vi "UMLEditor Main.vi"(1 "StartProject":string, 3 "StartTarget":string) -> ()   [LabVIEW 2012] (continued)
            n1875 = call <resource>:"UMLEditor getDiagramInfo.vi"("localVariables"=w4885, "error in (no error)"=w4887) -> ("saveDir"=w4893:path, "error out"=w4886:errorcluster)  [unwired: 16 out]
            n1876 = File Dialog(6:"*.txt" ("pattern"), 7:"Select script file to start executing" ("prompt"), 11:w4893) -> (1:w4890:bool, 2:w4891:bool, 3:w4888:path)  [unwired: 1 in, 4 out]
            n1877 = Compound Arithmetic op=AND(w4891, invert w4890) -> (invert w4889:bool)
          }
          frame Default {
            n1878 = Equal?(x=w4902, y=UMLEditor_statesType."ExecuteCommand" ("state")) -> (x = y?=w4901:bool)
            n1879 = call <resource>:"UMLEditor createWizardScriptFile.vi"("localVariables"=w4899, "OnlySelectedNode(False)"=w4901, "error in (no error)"=w4904) -> ("localVariables"=w4898:T7, "pathToScriptFile"=w4903:path, "Cancelled"=w4895:bool, "error out"=w4897:errorcluster)  [unwired: 13 out]
          }
        }
        n1880 = call <resource>:"CommonVIs_UmlOpenVIRef.vi"("error in"=w4879) -> ("error out"=w4873:errorcluster, "ProjectNameOut"=w4870:string)  [unwired: 3 in, 6 out]
        n1881 = call <resource>:"GDSProject_GetProjects.vi"("GetProjectRefByName"=w4870, "error in (no error)"=w4873) -> ("Projects"=w4872:string[], "Project Refnum"=w4869:refnum<vi>)  [unwired: 1 in, 15 out]
        n1882 = Search 1D Array(1D array=w4872, element=w4870) -> (index of element=w4871:i32)  [unwired: 1 out]
        n1883 = property on="Project" class="Ring (strict)"("Strings []"=w4872, "Value"=w4871) -> ()  [unwired: 2 in, 2 out]
        n1884 = property class="Project"(reference=w4869) -> (reference out=w4866:refnum<vi>, error out=w4867:errorcluster, "Path"=w4865:path)  [unwired: 1 in]
        n1885 = call <resource>:"GetRelativePathOption.vi"() -> ("UseProjectFolderAsBasePath"=w4868:bool)  [unwired: 1 in, 18 out]
        n1886 = Strip Path(path=w4865) -> (stripped path=w4862:path)  [unwired: 1 out]
        n1887 = Close Reference(reference=w4866, error in (no error)=w4867) -> (error out=w4861:errorcluster)
        n1888 = call <resource>:"File_ApplicationPaths.vi"("PathName"=UMLEditor_StoredPathes."LastSearchPath" ("UMLPathes"), "Path In"=w4862, "Method (Get Path)"=File_StoredPathesActions."Set Path") -> ()  [unwired: 1 in, 16 out]
        n1889 = case shown="True" w4868 {
          tunnel: w4862 -> [_ w4881]
          tunnel: w4861 -> [_ _]
          frame False {
          }
          frame True {
            n1890 = call <resource>:"File_ApplicationPaths.vi"("PathName"=UMLEditor_StoredPathes."ClassBasePath" ("UMLPathes"), "Path In"=w4881, "Method (Get Path)"=File_StoredPathesActions."Set Path") -> ()  [unwired: 1 in, 16 out]
          }
        }
      }
      frame "ClassReversedEngineering".."StateReversedEngineering" {
        n1891 = case shown="\"ClassReversedEngineering\", Default" w4909 {
          tunnel: w4916 -> [w4931 w4970 w4990]
          tunnel: [w4920 w4969 w4984] -> w4914
          tunnel: [w4923 w4968 w4990] -> w4913
          tunnel: [w4919 w4967 w4983] -> w4911
          tunnel: [enum32{"Class", "Sequence", "UseCase", "State"}."State" ("toolTab") enum32{"Class", "Sequence", "UseCase", "State"}."Class" ("toolTab") w4996] -> w4908
          tunnel: [diagramType."State" ("diagramType") diagramType."Class" ("diagramType") w4985] -> w4907
          tunnel: w4906 -> [w4918 w4963 w4986]
          tunnel: [w4918 w4964 w4986] -> w4905
          frame "StateReversedEngineering" {
            (unwired) T58."existing file" ("select mode (2)")
            n1892 = Unbundle By Name(w4918) -> ("grid"=w4921:refnum<class "Grid.lvclass">, "graphics"=w4922:refnum<class "Graphics.lvclass">)
            n1893 = File Dialog(4:"VIs" ("pattern label"), 6:"*.vi" ("pattern"), 7:"Select VI(containing a state machine) for analysing" ("prompt")) -> (1:w4927:bool, 3:w4926:path)  [unwired: 1 in, 5 out]
            n1894 = Bundle By Name(cluster=T32 {"VI-Path"=path "", "ShowOption"=enum."Show Relative Path"} ("StateDiagramData"), "VI-Path"=w4926) -> (w4924:T32)
            n1895 = case shown="True" w4927 {
              selector: w4927 -> [_ w4949]
              tunnel: w4931 -> [w4943 w4948]
              tunnel: w4924 -> [w4942 _]
              tunnel: [w4935 w4948] -> w4923
              tunnel: w4922 -> [w4939 _]
              tunnel: w4921 -> [w4938 _]
              tunnel: [w4934 w4949] -> w4920
              tunnel: [w4933 _] -> w4919
              frame False {
                n1896 = call <resource>:"StateDiagramGraph_Create.vi"("StateDiagramData"=w4942, "error in (no error)"=w4943) -> ("reference out"=w4941:refnum<class "StateDiagramGraph.lvclass">, "error out"=w4940:errorcluster)  [unwired: 2 in, 14 out]
                n1897 = call-dynamic "HandleRightClickMenuOption.vi"("reference"=w4941, "MenuOption"="Create New Diagram", "graphics"=w4939, "grid"=w4938, "error in (no error)"=w4940) -> ("reference out"=w4933:refnum<class "StateDiagramGraph.lvclass">, "Cancel"=w4934:bool, "error out"=w4936:errorcluster)  [unwired: 12 in]
                n1898 = case shown="True" w4934 {
                  tunnel: w4933 -> [_ w4947]
                  tunnel: w4936 -> [w4944 w4946]
                  tunnel: [w4944 w4945] -> w4935
                  frame False {
                  }
                  frame True {
                    n1899 = call-dynamic "Destroy.vi"("reference"=w4947, "error in (no error)"=w4946) -> ("error out"=w4945:errorcluster)  [unwired: 16 in, 1 out]
                  }
                }
              }
              frame True {
              }
            }
          }
          frame "ClassReversedEngineering", Default {
            n1900 = Unbundle By Name(w4963) -> ("XMI_Import"=w4951:bool, "Action"=w4960:string)
            n1901 = String To Path(string=w4960) -> (path=w4953:path)
            n1902 = File/Directory Info(path=w4953) -> (size=w4959:i64)  [unwired: 1 in, 6 out]
            n1903 = call <vilib>:"Librarian Get Info.vi"("path"=w4953) -> ("file information"=w4957:T62)  [unwired: 1 in, 9 out]
            n1904 = Unbundle By Name(w4957) -> ("size"=w4956:i32)
            n1905 = Greater Than 0?(x=w4959) -> (x > 0?=w4958:bool)
            n1906 = Greater Than 0?(x=w4956) -> (x > 0?=w4955:bool)
            n1907 = Equal?(x=w4960, y="WholeProject") -> (x = y?=w4961:bool)
            n1908 = Or(x=w4958, y=w4955) -> (x .or. y?=w4954:bool)
            n1909 = case shown="True" w4954 {
              tunnel: w4970 -> [w4976 w4982]
              tunnel: [w4975 w4981] -> w4969
              tunnel: [w4974 w4980] -> w4968
              tunnel: [w4973 w4979] -> w4967
              tunnel: w4961 -> [w4972 _]
              tunnel: w4953 -> [_ w4978]
              tunnel: w4951 -> [w4971 w4977]
              frame False {
                n1910 = call <resource>:"UMLEditor reversedEngineering.vi"("AddProjectClasses"=w4972, "XMI Import"=w4971, "error in (no error)"=w4976) -> ("cancel"=w4975:bool, "newCLassDiagram"=w4973:refnum<class "Graph.lvclass">, "error out"=w4974:errorcluster)  [unwired: 1 in, 13 out]
              }
              frame True {
                n1911 = call <resource>:"UMLEditor reversedEngineering.vi"("ClassToAnalyse/XMI File To Read"=w4978, "XMI Import"=w4977, "error in (no error)"=w4982) -> ("cancel"=w4981:bool, "newCLassDiagram"=w4979:refnum<class "Graph.lvclass">, "error out"=w4980:errorcluster)  [unwired: 1 in, 13 out]
              }
            }
            n1912 = Bundle By Name(cluster=w4963, "Action"="", "XMI_Import"=FALSE) -> (w4964:T7)
          }
          frame "PlugInReverseEngineering" {
            n1913 = call <resource>:"File_ApplicationPaths.vi"("PathName"=UMLEditor_StoredPathes."RevPlugInPath" ("UMLPathes")) -> ("Path Out"=w4987:path)  [unwired: 3 in, 15 out]
            n1914 = Open VI Reference(type specifier VI Refnum (for type only)=refnum<vi> refnum, vi path=w4987, error in (no error)=w4990) -> (vi reference=w4994:refnum<vi>, error out=w4993:errorcluster)  [unwired: 3 out]
            n1915 = call-by-ref "?"(reference=w4994, error in=w4993) -> (reference out=w4992:refnum<vi>, error out=w4991:errorcluster, "reference"=w4983:refnum<class "Graph.lvclass">, "cancelled"=w4984:bool, "diagramType"=w4985:T11)  [unwired: 8 in, 1 out]
            n1916 = case shown="\"Class\", Default" w4985 {
              tunnel: [enum32{"Class", "Sequence", "UseCase", "State"}."Class" ("toolTab") enum32{"Class", "Sequence", "UseCase", "State"}."Sequence" ("toolTab") enum32{"Class", "Sequence", "UseCase", "State"}."State" ("toolTab") enum32{"Class", "Sequence", "UseCase", "State"}."UseCase" ("toolTab")] -> w4996
              frame "Class", Default {
              }
              frame "Sequency" {
              }
              frame "State" {
              }
              frame "UseCase" {
              }
            }
            n1917 = Close Reference(reference=w4992, error in (no error)=w4991) -> (error out=w4989:errorcluster)
            n1918 = call <vilib>:"Simple Error Handler.vi"("error in (no error)"=w4989) -> ()  [unwired: 1 in, 8 out]
          }
        }
        n1919 = case shown="False" w4914 {
          tunnel: w4913 -> [w5015 w5040]
          tunnel: [w5021 w5040] -> w4915
          tunnel: [w5019 w5038] -> w4912
          tunnel: w4911 -> [w5016 _]
          tunnel: [UMLEditor_statesType."Repaint" ("state") UMLEditor_statesType."Idle" ("state")] -> w4910
          tunnel: w4908 -> [w5001 _]
          tunnel: w4907 -> [w5009 _]
          tunnel: w4905 -> [w5004 w5038]
          frame False {
            n1920 = Unbundle By Name(w5004) -> ("diagrams"=w5032:T39)
            n1921 = Unbundle By Name(w5004) -> ("grid"=w5012:refnum<class "Grid.lvclass">, "graphics"=w5013:refnum<class "Graphics.lvclass">)
            n1922 = for {
              tunnel: w5032 -> [w5037] mode=indexing
              tunnel: "Untitled %d" -> [w5035]
              tunnel: [w5034] -> w5030 mode=indexing
              n1923 = Unbundle By Name(w5037) -> ("name"=w5036:string)
              n1924 = Scan From String(format string=w5035, input string=w5036) -> (output 1=w5034:i32)  [unwired: 2 in, 4 out]
            }
            n1925 = property on="toolTab" class="TabCtl (strict)"("Value"=w5001) -> ()  [unwired: 2 in, 2 out]
            n1926 = Array Max & Min(array=w5030) -> (max value=w5029:i32)  [unwired: 3 out]
            n1927 = call-dynamic "draw.vi"("reference"=w5016, "graphics"=w5013, "grid"=w5012, "error in (no error)"=w5015, "SelectedNodes"=refnum<class "AbstractNode.lvclass">[] [], "HideOverLays(False)"=FALSE) -> ("NodesBounds"=w5011:T13, "error out"=w5014:errorcluster)  [unwired: 10 in, 2 out]
            n1928 = Increment(x=w5029) -> (x+1=w5027:i32)
            n1929 = Bundle By Name(cluster=w5004, "NodesBounds"=w5011) -> (w5007:T7)
            n1930 = Format Into String(format string="Untitled %d", w5027) -> (resulting string=w5017:string)  [unwired: 2 in, 1 out]
            n1931 = property on="Diagram" class="Ring (strict)"("Tip Strip"=w5017) -> ()  [unwired: 2 in, 2 out]
            n1932 = Unbundle By Name(w5007) -> ("menu"=w5006:refnum<k9>)
            n1933 = property on="toolTab" class="TabCtl (strict)"("Disabled"=u8 0) -> ()  [unwired: 2 in, 2 out]
            n1934 = call <resource>:"UMLEditor addDiagram.vi"("graph"=w5016, "diagramType"=w5009, "name"=w5017, "saveDir"=path "", "unsaved(False)"=TRUE, "error in (no error)"=w5014, "localVariablesIn"=w5007) -> ("localVariablesOut"=w5005:T7, "error out"=w5025:errorcluster)  [unwired: 11 out]
            n1935 = local write "Diagram"(0) -> ()
            n1936 = call <resource>:"UMLEditor menuUpdates.vi"("menu"=w5006, "menuAction"=UMLEditor_MenuActionType."EnableSave", "error in (no error)"=w5025) -> ("error out"=w5020:errorcluster)  [unwired: 3 in, 13 out]
            n1937 = property on="Picture" class="Pict"("Visible"=TRUE) -> ()  [unwired: 2 in, 2 out]
            n1938 = call <resource>:"UMLEditor setDiagramInfo.vi"("error in (no error)"=w5020, "localVariablesIn"=w5005, "action"=enum16{"Name/Dir", "Unsaved", "Saved"}."Unsaved") -> ("localVariablesOut"=w5019:T7, "error out"=w5021:errorcluster)  [unwired: 2 in, 13 out]
          }
          frame True {
          }
        }
      }
      frame "PanAndRepaint" {
        n1939 = Unbundle By Name(w5060) -> ("graphics"=w5059:refnum<class "Graphics.lvclass">, "SelectedNodes"=w5058:refnum<class "AbstractNode.lvclass">[])
        n1940 = Index Array(array=w5058) -> (element=w5057:refnum<class "AbstractNode.lvclass">)  [unwired: 1 in]
        n1941 = To More Specific Class(target class=refnum<class "RectangularNode.lvclass"> refnum ("reference"), reference=w5057, error in=w5055) -> (specific class reference=w5054:refnum<class "RectangularNode.lvclass">, error out=w5053:errorcluster)
        n1942 = call <resource>:"getScreenBounds.vi"("reference"=w5059) -> ("bounds"=w5048:T13)  [unwired: 1 in, 17 out]
        n1943 = call-dynamic "getBounds.vi"("reference"=w5054, "error in (no error)"=w5053) -> ("bounds"=w5042:T13, "error out"=w5044:errorcluster)  [unwired: 15 in, 1 out]
        n1944 = Unbundle By Name(w5048) -> ("width"=w5043:dbl, "height"=w5041:dbl)
        n1945 = property on="Picture" class="Pict"() -> ("Origin:Left"=w5050:i16, "Origin:Top"=w5049:i16)  [unwired: 2 in, 2 out]
        n1946 = Unbundle By Name(w5042) -> ("x"=w5052:dbl, "y"=w5051:dbl)
        n1947 = In Range and Coerce(upper limit=w5043, x=w5052, lower limit=w5050) -> (In Range?=w5047:bool)  [unwired: 1 out]
        n1948 = In Range and Coerce(upper limit=w5041, x=w5051, lower limit=w5049) -> (In Range?=w5046:bool)  [unwired: 1 out]
        n1949 = And(x=w5047, y=w5046) -> (x .and. y?=w5045:bool)
        n1950 = case shown="False" w5045 {
          tunnel: w5043 -> [w5075 _]
          tunnel: w5042 -> [w5073 _]
          tunnel: w5041 -> [w5068 _]
          frame False {
            w5062 = 0.0 ("y")
            n1951 = call <resource>:"Rectangel GetRectInfo.vi"("bounds"=w5073) -> ("centerX"=w5072:dbl, "centerY"=w5070:dbl)  [unwired: 14 in, 3 out]
            n1952 = Divide(x=w5075, y=2.0) -> (x/y=w5071:dbl)
            n1953 = Divide(x=w5068, y=2.0) -> (x/y=w5067:dbl)
            n1954 = Subtract(x=w5072, y=w5071) -> (x-y=w5066:dbl)
            n1955 = Subtract(x=w5070, y=w5067) -> (x-y=w5064:dbl)
            n1956 = Max & Min(x=w5066, y=w5062) -> (max(x,y)=w5065:dbl)  [unwired: 1 out]
            n1957 = Max & Min(x=w5064, y=w5062) -> (max(x,y)=w5063:dbl)  [unwired: 1 out]
            n1958 = property on="Picture" class="Pict"("Origin:Left"=w5065, "Origin:Top"=w5063) -> ()  [unwired: 2 in, 2 out]
          }
          frame True {
          }
        }
      }
      frame "Repaint" {
        n1959 = Unbundle By Name(w5079) -> ("selcted"=w5094:T9)
        n1960 = call <resource>:"UMLEditor getDiagramInfo.vi"("localVariables"=w5079, "error in (no error)"=w5092) -> ("diagramType"=w5084:T11, "error out"=w5086:errorcluster)  [unwired: 16 out]
        n1961 = case shown="\"Node\", \"Edge\"" w5094 {
          tunnel: [w5104 UMLEditor_MenuActionType."enablePropDel" ("menuAction")] -> w5093
          tunnel: w5084 -> [w5103 _]
          frame "None", Default {
            n1962 = case shown="Default" w5103 {
              tunnel: [UMLEditor_MenuActionType."enablePropDisDel" ("menuAction") UMLEditor_MenuActionType."disablePropDel" ("menuAction")] -> w5104
              frame "State" {
              }
              frame Default {
              }
            }
          }
          frame "Node", "Edge" {
          }
        }
        n1963 = Equal?(x=w5084, y=diagramType."None") -> (x = y?=w5090:bool)
        n1964 = Unbundle By Name(w5079) -> ("menu"=w5077:refnum<k9>)
        n1965 = call <resource>:"UMLEditor ToolsMenuUpdates.vi"("menu"=w5077, "diagramType"=w5084, "error in (no error)"=w5086) -> ("error out"=w5085:errorcluster)  [unwired: 2 in, 14 out]
        n1966 = call <resource>:"UMLEditor menuUpdates.vi"("menu"=w5077, "menuAction"=w5093, "error in (no error)"=w5085) -> ("error out"=w5095:errorcluster)  [unwired: 3 in, 13 out]
        n1967 = call <resource>:"UMLEditor updateDiagramsInfo.vi"("localVariables"=w5079, "error in (no error)"=w5095) -> ("diagramNames"=w5099:string[], "index"=w5083:i32, "currentIsUnsaved"=w5078:bool, "notSavedBefore"=w5096:bool, "error out"=w5076:errorcluster)  [unwired: 13 out]
        n1968 = while {
          shift-right: [w5101] -> _
          shift-left: _ -> [w5100]
          tunnel: w5083 -> [w5101]
          tunnel: [w5100] -> w5082
          stop <- TRUE stop-if-true
        }
        n1969 = property on="Diagram" class="Ring (strict)"() -> ("Strings []"=w5098:string[])  [unwired: 2 in, 2 out]
        n1970 = Not Equal?(x=w5082, y=w5083) -> (x != y?=w5080:bool)
        n1971 = Not Equal?(x=w5099, y=w5098) -> (x != y?=w5097:bool)
        n1972 = Or(x=w5080, y=w5097) -> (x .or. y?=w5081:bool)
        n1973 = case shown="True" w5081 {
          tunnel: w5099 -> [_ w5112]
          tunnel: w5083 -> [_ w5110]
          tunnel: w5078 -> [_ w5109]
          tunnel: w5096 -> [_ w5111]
          tunnel: w5077 -> [_ w5108]
          frame False {
          }
          frame True {
            n1974 = Compound Arithmetic op=AND(w5109, invert w5111) -> ()  [unwired: 1 out]
            n1975 = property on="Diagram" class="Ring (strict)"("Strings []"=w5112) -> ()  [unwired: 2 in, 2 out]
            n1976 = local write "Diagram"(w5110) -> ()
            n1977 = case shown="True" w5109 {
              tunnel: w5108 -> [w5113 w5115]
              frame True {
                n1978 = call <resource>:"UMLEditor menuUpdates.vi"("menu"=w5113, "menuAction"=UMLEditor_MenuActionType."EnableSave") -> ()  [unwired: 4 in, 14 out]
              }
              frame False {
                n1979 = call <resource>:"UMLEditor menuUpdates.vi"("menu"=w5115, "menuAction"=UMLEditor_MenuActionType."DiableSave") -> ()  [unwired: 4 in, 14 out]
              }
            }
          }
        }
        n1980 = Select(t=UMLEditor_statesType."Idle", s=w5090, f=UMLEditor_statesType."PaintComponent" ("state")) -> (s? t:f=w5088:T8)
      }
      frame "PaintComponent" {
        n1981 = Unbundle By Name(w5129) -> ("menu"=w5128:refnum<k9>)
        n1982 = Unbundle By Name(w5129) -> ("selcted"=w5138:T9, "selectedEdge"=w5148:refnum<class "AbstractEdge.lvclass">, "SelectedNodes"=w5123:refnum<class "AbstractNode.lvclass">[], "ObjectHotspots"=w5122:T18[], "NodesBounds"=w5136:T13)
        n1983 = Unbundle By Name(w5129) -> ("newSelected"=w5145:bool, "zoom"=w5152:dbl, "grid"=w5146:refnum<class "Grid.lvclass">, "offset"=w5139:T12, "graphics"=w5142:refnum<class "Graphics.lvclass">, "hideGrid"=w5151:bool)  [unwired: 1 out]
        n1984 = Unbundle By Name(w5129) -> ("butDwn"=w5132:bool)
        n1985 = Unbundle By Name(w5129) -> ("ResizePanelInProgress"=w5133:bool)
        n1986 = call <resource>:"UMLEditor getDiagramInfo.vi"("localVariables"=w5129, "error in (no error)"=w5150) -> ("graph"=w5130:refnum<class "Graph.lvclass">, "error out"=w5140:errorcluster)  [unwired: 16 out]
        n1987 = case shown="False" w5145 {
          tunnel: w5152 -> [w5168 _]
          tunnel: w5151 -> [w5169 _]
          tunnel: w5130 -> [w5184 w5216]
          tunnel: [w5183 w5216] -> w5149
          tunnel: [w5182 w5217] -> w5131
          tunnel: w5140 -> [w5181 w5217]
          tunnel: w5142 -> [w5180 _]
          tunnel: w5146 -> [w5179 _]
          tunnel: w5141 -> [_ _]
          tunnel: w5139 -> [w5178 _]
          tunnel: [w5171 w5215] -> w5137
          tunnel: w5136 -> [w5172 w5215]
          tunnel: w5123 -> [w5164 _]
          tunnel: [w5163 w5212] -> w5120
          tunnel: w5122 -> [_ w5214]
          frame False {
            n1988 = call <resource>:"resetPicture.vi"("reference"=w5180, "error in (no error)"=w5181) -> ("reference out"=w5177:refnum<class "Graphics.lvclass">, "error out"=w5176:errorcluster)  [unwired: 16 out]
            n1989 = call <resource>:"getScreenBounds.vi"("reference"=w5177, "error in (no error)"=w5176) -> ("reference out"=w5175:refnum<class "Graphics.lvclass">, "bounds"=w5173:T13, "ZoomChanged"=w5165:bool, "error out"=w5174:errorcluster)  [unwired: 14 out]
            n1990 = Less?(x=w5168, y=0.5) -> (x < y?=w5166:bool)
            n1991 = Or(x=w5166, y=w5169) -> (x .or. y?=w5170:bool)
            n1992 = case shown="False" w5170 {
              tunnel: w5179 -> [w5210 _]
              tunnel: w5168 -> [_ _]
              tunnel: [w5209 w5211] -> w5185
              tunnel: w5178 -> [_ _]
              tunnel: w5175 -> [w5208 _]
              tunnel: w5174 -> [w5207 w5211]
              tunnel: w5173 -> [w5202 _]
              tunnel: w5172 -> [w5206 _]
              tunnel: w5165 -> [w5191 _]
              frame False {
                w5186 = 500
                w5204 = 50
                w5201 = 0.0 ("x")
                n1993 = Unbundle By Name(w5206) -> ("width"=w5205:dbl, "height"=w5203:dbl)
                n1994 = Unbundle By Name(w5202) -> ("width"=w5200:dbl, "height"=w5199:dbl)
                n1995 = property on="Picture" class="Pict"() -> ("Origin:Left"=w5194:i16, "Origin:Top"=w5193:i16)  [unwired: 2 in, 2 out]
                n1996 = Add(x=w5204, y=w5203) -> (x+y=w5195:dbl)
                n1997 = Add(x=w5204, y=w5205) -> (x+y=w5198:dbl)
                n1998 = Add(x=w5194, y=w5200) -> (x+y=w5197:dbl)
                n1999 = Add(x=w5193, y=w5199) -> (x+y=w5196:dbl)
                n2000 = Max & Min(x=w5198, y=w5197) -> (max(x,y)=w5190:dbl)  [unwired: 1 out]
                n2001 = Max & Min(x=w5195, y=w5196) -> (max(x,y)=w5188:dbl)  [unwired: 1 out]
                n2002 = Add(x=w5186, y=w5188) -> (x+y=w5187:dbl)
                n2003 = Add(x=w5186, y=w5190) -> (x+y=w5189:dbl)
                n2004 = Bundle(cluster=w5202, "x"=w5201, "y"=w5201, "width"=w5189, "height"=w5187) -> (w5192:T13)
                n2005 = call-dynamic "draw.vi"("reference"=w5210, "graphics"=w5208, "bounds"=w5192, "ForceRedrawGrid"=w5191, "error in (no error)"=w5207) -> ("error out"=w5209:errorcluster)  [unwired: 13 in, 1 out]
              }
              frame True {
              }
            }
            n2006 = call-dynamic "draw.vi"("reference"=w5184, "graphics"=w5180, "grid"=w5179, "error in (no error)"=w5185, "SelectedNodes"=w5164, "HideOverLays(False)"=FALSE) -> ("reference out"=w5183:refnum<class "Graph.lvclass">, "NodesBounds"=w5171:T13, "HotSpots"=w5163:T18[], "error out"=w5182:errorcluster)  [unwired: 10 in]
          }
          frame True {
            n2007 = for {
              tunnel: w5214 -> [w5219] mode=indexing
              shift-right: [w5218] -> w5212
              shift-left: T18[] [] -> [w5220]
              n2008 = Unbundle By Name(w5219) -> ("Function"=w5221:T19)
              n2009 = case shown="\"Expand\", \"Collaps\"" w5221 {
                tunnel: w5220 -> [w5222 w5225]
                tunnel: w5219 -> [_ w5224]
                tunnel: [w5222 w5223] -> w5218
                frame Default {
                }
                frame "Expand", "Collaps" {
                  n2010 = Build Array (concatenate)(w5225, w5224) -> (w5223:T18[])
                }
              }
            }
          }
        }
        n2011 = Compound Arithmetic op=AND(invert w5132, invert w5133) -> (w5127:bool)
        n2012 = call <resource>:"UMLEditor_GraphMemory.vi"("GraphIn"=w5130) -> ()  [unwired: 1 in, 18 out]
        n2013 = call <resource>:"updateScreen.vi"("reference"=w5142, "error in (no error)"=w5131) -> ("reference out"=w5126:refnum<class "Graphics.lvclass">, "error out"=w5143:errorcluster)  [unwired: 16 out]
        n2014 = case shown="True" w5127 {
          tunnel: w5131 -> [w5156 w5161]
          tunnel: [w5156 w5160] -> _
          tunnel: w5130 -> [_ w5159]
          tunnel: w5128 -> [_ w5157]
          frame False {
          }
          frame True {
            n2015 = call <resource>:"UndoEngine.vi"("reference"=w5159, "Action"=enum16{"TakeSnapshot", "Undo", "Redo"}."TakeSnapshot", "error in (no error)"=w5161, "menu"=w5157) -> ("error out"=w5160:errorcluster)  [unwired: 4 in, 11 out]
          }
        }
        n2016 = case shown="\"None\", Default" w5138 {
          tunnel: [w5228 w5236 w5258] -> w5119
          tunnel: w5149 -> [_ w5239 w5264]
          tunnel: w5143 -> [w5228 w5238 w5263]
          tunnel: w5148 -> [_ w5232 _]
          tunnel: [TRUE w5231 w5260] -> w5134
          tunnel: w5142 -> [_ w5235 w5257]
          tunnel: w5123 -> [_ _ w5262]
          tunnel: w5126 -> [_ w5230 w5253]
          tunnel: [w5226 w5229 w5254] -> w5121
          tunnel: w5120 -> [w5226 w5229 w5252]
          frame "None", Default {
          }
          frame "Edge" {
            n2017 = call-dynamic "getEdges.vi"("reference"=w5239, "error in (no error)"=w5238) -> ("edges"=w5237:refnum<class "AbstractEdge.lvclass">[], "error out"=w5234:errorcluster)  [unwired: 15 in, 1 out]
            n2018 = Search 1D Array(1D array=w5237, element=w5232) -> (index of element=w5233:i32)  [unwired: 1 in]
            n2019 = Less Than 0?(x=w5233) -> (x < 0?=w5231:bool)
            n2020 = case shown="0, Default" w5233 {
              tunnel: [w5250 w5251] -> w5236
              tunnel: w5235 -> [w5249 _]
              tunnel: w5234 -> [w5248 w5251]
              tunnel: w5232 -> [w5247 _]
              tunnel: w5230 -> [w5240 _]
              frame 0, Default {
                n2021 = call-dynamic "getConnectionPoints.vi"("reference"=w5247, "error in (no error)"=w5248) -> ("reference out"=w5243:refnum<class "AbstractEdge.lvclass">, "connectionPoints"=w5246:T12[], "error out"=w5245:errorcluster)  [unwired: 15 in]
                n2022 = call-dynamic "GetTextPositions.vi"("reference"=w5243, "GraphicsRef"=w5240, "error in (no error)"=w5245) -> ("connectionPoints"=w5241:T12[], "error out"=w5244:errorcluster)  [unwired: 14 in, 1 out]
                n2023 = Build Array (concatenate)(w5246, w5241) -> (w5242:T12[])
                n2024 = call <resource>:"UMLEditor drawGrabbers.vi"("graphics"=w5249, "points"=w5242, "error in (no error)"=w5244) -> ("error out"=w5250:errorcluster)  [unwired: 16 out]
              }
              frame -1 {
              }
            }
          }
          frame "Node" {
            n2025 = Array Size(array=w5262) -> (size(s)=w5261:i32)
            n2026 = for {
              tunnel: w5264 -> [w5275]
              tunnel: w5262 -> [w5271] mode=indexing
              shift-right: [w5270] -> w5259
              shift-left: w5263 -> [_]
              shift-right: [w5268] -> w5256
              shift-left: T12[] [] -> [w5269]
              shift-right: [w5267] -> w5254
              shift-left: w5252 -> [w5266]
              tunnel: w5253 -> [w5265]
              n2027 = call-dynamic "getNodes.vi"("reference"=w5275) -> ("nodes"=w5274:refnum<class "AbstractNode.lvclass">[], "error out"=w5273:errorcluster)  [unwired: 16 in, 1 out]
              n2028 = Search 1D Array(1D array=w5274, element=w5271) -> (index of element=w5272:i32)  [unwired: 1 in]
              n2029 = case shown="0, Default" w5272 {
                tunnel: [w5276 w5287] -> w5270
                tunnel: w5273 -> [w5283 w5287]
                tunnel: w5271 -> [w5278 _]
                tunnel: w5269 -> [w5284 w5286]
                tunnel: [w5282 w5286] -> w5268
                tunnel: [w5281 w5285] -> w5267
                tunnel: w5266 -> [w5280 w5285]
                tunnel: w5265 -> [_ _]
                frame 0, Default {
                  n2030 = call-dynamic "GetGrabberPositions.vi"("reference"=w5278, "error in (no error)"=w5283) -> ("GrabberPositions"=w5279:T12[], "HotSpots"=w5277:T18[], "error out"=w5276:errorcluster)  [unwired: 14 in, 1 out]
                  n2031 = Build Array (concatenate)(w5280, w5277) -> (w5281:T18[])
                  n2032 = Build Array (concatenate)(w5284, w5279) -> (w5282:T12[])
                }
                frame -1 {
                }
              }
            }
            n2033 = Less Or Equal To 0?(x=w5261) -> (x <= 0?=w5260:bool)
            n2034 = call <resource>:"UMLEditor drawGrabbers.vi"("graphics"=w5257, "points"=w5256, "error in (no error)"=w5259) -> ("error out"=w5258:errorcluster)  [unwired: 16 out]
          }
        }
        n2035 = Bundle By Name(cluster=w5129, "newSelected"=FALSE, "NodesBounds"=w5137) -> (w5135:T7)
        n2036 = case shown="True" w5134 {
          tunnel: [w5288 w5290] -> w5124
          tunnel: w5135 -> [w5288 w5291]
          frame False {
          }
          frame True {
            n2037 = Bundle By Name(cluster=w5291, "selcted"=UMLEditor_tooltype."None") -> (w5290:T7)
          }
        }
        n2038 = Tick Count (ms)() -> (millisecond timer value=w5117:u32)
        n2039 = case shown="True" w5118 {
          tunnel: w5119 -> [_ _]
          tunnel: w5117 -> [_ w5153]
          frame False {
          }
          frame True {
            n2040 = Tick Count (ms)() -> (millisecond timer value=w5155:u32)
            n2041 = Subtract(x=w5155, y=w5153) -> (x-y=→"Time":u32)
          }
        }
        n2042 = Bundle By Name(cluster=w5124, "ObjectHotspots"=w5121) -> (w5125:T7)
      }
      frame "AutoPlace" {
        n2043 = call <resource>:"ArrangeNodes Main.vi"("localVariablesOut"=w5294) -> ("Cancel"=w5292:bool)  [unwired: 1 in, 17 out]
        n2044 = case shown="False" w5292 {
          tunnel: w5296 -> [w5299 w5305]
          tunnel: [w5299 w5304] -> w5295
          tunnel: [w5298 w5301] -> w5293
          tunnel: w5294 -> [w5298 w5303]
          frame True {
          }
          frame False {
            n2045 = call <resource>:"UMLEditor setDiagramInfo.vi"("error in (no error)"=w5305, "localVariablesIn"=w5303, "action"=enum16{"Name/Dir", "Unsaved", "Saved"}."Unsaved") -> ("localVariablesOut"=w5302:T7, "error out"=w5304:errorcluster)  [unwired: 2 in, 13 out]
            n2046 = Bundle By Name(cluster=w5302, "modified"=TRUE) -> (w5301:T7)
          }
        }
      }
      frame "ExecuteCommand" {
        n2047 = Unbundle By Name(w5309) -> ("FlattenCommandSettings.Command"=w5317:T16, "FlattenCommandSettings.CommandData"=w5311:variant, "selcted"=w5316:T9, "SelectedNodes"=w5313:refnum<class "AbstractNode.lvclass">[])  [unwired: 1 out]
        n2048 = Unbundle By Name(w5309) -> ("graphics"=w5308:refnum<class "Graphics.lvclass">, "grid"=w5307:refnum<class "Grid.lvclass">)
        n2049 = call <resource>:"UMLEditor getDiagramInfo.vi"("localVariables"=w5309, "error in (no error)"=w5315) -> ("graph"=w5310:refnum<class "Graph.lvclass">, "error out"=w5314:errorcluster)  [unwired: 16 out]
        n2050 = case shown="\"OpenClassAttribute\"" w5317 {
          tunnel: [w5330 UMLEditor_statesType."Idle" ("state") UMLEditor_statesType."Idle" ("state") UMLEditor_statesType."CreateScript" ("state") UMLEditor_statesType."Idle" ("state") UMLEditor_statesType."Idle" ("state") w5538 UMLEditor_statesType."Idle" ("state")] -> w5319
          tunnel: w5314 -> [w5329 w5411 w5416 w5441 w5447 w5464 w5556 w5582]
          tunnel: [w5326 w5411 w5416 w5441 w5446 w5462 w5556 w5580] -> w5318
          tunnel: w5316 -> [w5328 _ _ _ _ _ _ _]
          tunnel: w5313 -> [w5327 _ _ _ _ _ w5557 w5581]
          tunnel: w5309 -> [w5325 w5413 w5429 w5439 w5456 w5469 w5537 w5584]
          tunnel: [w5324 w5413 w5429 w5439 w5456 w5469 w5536 w5584] -> w5312
          tunnel: w5310 -> [w5323 _ _ _ _ _ _ _]
          tunnel: w5311 -> [_ w5414 w5430 w5443 w5457 w5470 _ _]
          tunnel: w5309 -> [w5322 _ _ _ _ _ _ _]
          tunnel: w5310 -> [_ _ _ _ _ _ _ w5583]
          tunnel: w5308 -> [w5321 _ _ _ _ _ _ _]
          tunnel: w5307 -> [w5320 _ _ _ _ _ _ _]
          frame "SyncUmlFromCode", Default {
            n2051 = case shown="\"Node\"" w5328 {
              tunnel: [UMLEditor_statesType."Repaint" ("state") UMLEditor_statesType."Repaint" ("state")] -> w5330
              tunnel: w5329 -> [w5333 w5357]
              tunnel: w5327 -> [_ w5359]
              tunnel: [w5333 w5362] -> w5326
              tunnel: w5325 -> [w5331 w5361]
              tunnel: [w5331 w5360] -> w5324
              tunnel: w5323 -> [_ w5354]
              tunnel: w5322 -> [_ _]
              tunnel: w5321 -> [_ w5353]
              tunnel: w5320 -> [_ w5352]
              frame "None", Default {
              }
              frame "Node" {
                n2052 = Index Array(array=w5359) -> (element=w5336:refnum<class "AbstractNode.lvclass">)  [unwired: 1 in]
                n2053 = To More Specific Class(target class=refnum<class "ClassNode.lvclass"> refnum ("reference"), reference=w5336) -> (specific class reference=w5335:refnum<class "ClassNode.lvclass">)  [unwired: 1 in, 1 out]
                n2054 = call-dynamic "getClassInfo.vi"("reference"=w5335, "error in (no error)"=w5357) -> ("methods(string)"=w5340:string, "attributes(string)"=w5347:string, "reference out"=w5355:refnum<class "ClassNode.lvclass">, "className"=w5351:string, "ClassPath"=w5358:path, "error out"=w5356:errorcluster)  [unwired: 8 in, 4 out]
                n2055 = call <resource>:"ReversedEngineering SyncUmlFromCode.vi"("SyncAction"=ReversedEngineering_SyncUmlFromCodeActions."GetAll", "ClassPath"=w5358, "NodeRef"=w5355, "GraphRef"=w5354, "error in (no error)"=w5356, "ClassName(needed for lllbs)"=w5351, "graphics"=w5353, "grid"=w5352) -> ("ClassName"=w5338:string, "attributes"=w5348:string, "methods"=w5346:string, "error out"=w5367:errorcluster)  [unwired: 4 in, 4 out]
                n2056 = Empty String/Path?(string/path=w5338) -> (empty?=w5337:bool)
                n2057 = Empty String/Path?(string/path=w5340) -> (empty?=w5350:bool)
                n2058 = Empty String/Path?(string/path=w5347) -> (empty?=w5349:bool)
                n2059 = Equal?(x=w5348, y=w5347) -> (x = y?=w5344:bool)
                n2060 = Equal?(x=w5346, y=w5340) -> (x = y?=w5345:bool)
                n2061 = And(x=w5350, y=w5349) -> (x .and. y?=w5342:bool)
                n2062 = And(x=w5344, y=w5345) -> (x .and. y?=w5343:bool)
                n2063 = Or(x=w5343, y=w5342) -> (x .or. y?=w5341:bool)
                n2064 = case shown="True" w5341 {
                  tunnel: w5367 -> [w5378 w5379]
                  tunnel: [w5377 FALSE ("CancelOut")] -> w5366
                  tunnel: [w5376 w5379] -> w5365
                  tunnel: [w5375 w5381] -> w5364
                  tunnel: [w5374 w5380] -> w5363
                  tunnel: w5348 -> [w5373 w5381]
                  tunnel: w5347 -> [w5372 _]
                  tunnel: w5346 -> [w5371 w5380]
                  tunnel: w5340 -> [w5370 _]
                  frame False {
                    n2065 = call <resource>:"UMLEditor UpdateMethodsAttributesDialog.vi"("OldAttributesIn"=w5372, "OldMethodsIn"=w5370, "New Attributes"=w5373, "New Methods"=w5371, "error in (no error)"=w5378) -> ("AttributesOut"=w5375:string, "MethodsOut"=w5374:string, "CancelOut"=w5377:bool, "error out"=w5376:errorcluster)  [unwired: 11 out]
                  }
                  frame True {
                  }
                }
                n2066 = Or(x=w5337, y=w5366) -> (x .or. y?=w5339:bool)
                n2067 = case shown="True" w5339 {
                  tunnel: w5365 -> [w5385 w5403]
                  tunnel: w5355 -> [w5389 _]
                  tunnel: w5364 -> [w5391 _]
                  tunnel: w5363 -> [w5394 _]
                  tunnel: [w5392 w5403] -> w5362
                  tunnel: w5361 -> [w5396 w5402]
                  tunnel: [w5395 w5402] -> w5360
                  tunnel: w5354 -> [w5384 _]
                  tunnel: w5338 -> [w5387 _]
                  frame False {
                    n2068 = call-dynamic "ExternalSetParam.vi"("reference"=w5389, "setParameter"=ExternalSetTypes."Name", "string"=w5387, "error in (no error)"=w5385) -> ("reference out"=w5388:refnum<class "ClassNode.lvclass">, "error out"=w5386:errorcluster)  [unwired: 14 in]
                    n2069 = call-dynamic "ExternalSetParam.vi"("reference"=w5388, "setParameter"=ExternalSetTypes."Attributes", "string"=w5391, "error in (no error)"=w5386) -> ("reference out"=w5399:refnum<class "ClassNode.lvclass">, "error out"=w5400:errorcluster)  [unwired: 14 in]
                    n2070 = call-dynamic "ExternalSetParam.vi"("reference"=w5399, "setParameter"=ExternalSetTypes."Methods", "string"=w5394, "error in (no error)"=w5400) -> ("error out"=w5383:errorcluster)  [unwired: 14 in, 1 out]
                    n2071 = call <resource>:"UMLEditor setDiagramInfo.vi"("error in (no error)"=w5383, "localVariablesIn"=w5396, "action"=enum16{"Name/Dir", "Unsaved", "Saved"}."Unsaved") -> ("localVariablesOut"=w5395:T7, "error out"=w5393:errorcluster)  [unwired: 2 in, 13 out]
                    n2072 = call-dynamic "layout.vi"("reference"=w5384, "error in (no error)"=w5393) -> ("error out"=w5392:errorcluster)  [unwired: 16 in, 1 out]
                  }
                  frame True {
                  }
                }
              }
            }
          }
          frame "OpenClass" {
            w5405 = "Refresh"  # Message
            w5409 = "Open class"  # Message
            n2073 = Variant To Data(type=path "", Variant=w5414) -> (data=w5407:path)  [unwired: 1 in, 1 out]
            n2074 = Path To String(path=w5407) -> (string=w5408:string)
            n2075 = call <resource>:"UMLEditor SendMessageToWizard.vi"("MessageType"=w5409, "MessageData"=w5408, "error in (no error)"=w5411) -> ("error out"=w5404:errorcluster)  [unwired: 1 in, 15 out]
            n2076 = call <resource>:"UMLEditor SendMessageToWizard.vi"("MessageType"=w5405, "AllowErrorPopup(True)"=FALSE, "error in (no error)"=w5404) -> ()  [unwired: 1 in, 16 out]
          }
          frame "OpenClassAttribute" {
            n2077 = Variant To Data(error in=w5416, type=path "", Variant=w5430) -> (data=w5426:path, error out=w5425:errorcluster)
            n2078 = call <resource>:"CreateReaderFromClass.vi"("ClassPath/LvClassRef"=w5426, "error in"=w5425) -> ("ClassReader"=w5424:refnum<class "ClassReader.lvclass">, "error out"=w5423:errorcluster)  [unwired: 16 out]
            n2079 = call-dynamic "GetAttributes.vi"("ClassReader in"=w5424, "OnlyGetReference"=TRUE ("OnlyGetPath"), "error in (no error)"=w5423) -> ("ClassReader out"=w5421:refnum<class "ClassReader.lvclass">, "ObjectAttributeReference"=w5418:refnum<vi>, "error out"=w5420:errorcluster)  [unwired: 14 out]
            n2080 = call-dynamic <resource>:"CleanUp.vi"("reference in"=w5421, "error in (no error)"=w5420) -> ("error out"=w5419:errorcluster)  [unwired: 17 out]
            n2081 = Not A Number/Path/Refnum?(number/path/refnum=w5418) -> (NaN/Path/Refnum?=w5417:bool)
            n2082 = case shown="False" w5417 {
              tunnel: [w5434 w5438] -> w5415
              tunnel: w5419 -> [w5433 w5438]
              tunnel: w5418 -> [w5432 _]
              frame False {
                n2083 = property class="VI"(reference=w5432, error in=w5433, "Front Panel.Open"=TRUE ("Front Panel Window:Open")) -> (reference out=w5435:refnum<vi>, error out=w5436:errorcluster)
                n2084 = Close Reference(reference=w5435, error in (no error)=w5436) -> (error out=w5434:errorcluster)
              }
              frame True {
              }
            }
            n2085 = case shown="Error" w5415 {
              frame No Error {
              }
              frame Error {
                n2086 = One Button Dialog(message="The file was not possible to open with this version of LabVIEW") -> ()  [unwired: 1 in, 1 out]
              }
            }
          }
          frame "CreateClass" {
            n2087 = Variant To Data(type=path "", Variant=w5443) -> ()  [unwired: 1 in, 2 out]
          }
          frame "OpenFile" {
            n2088 = Variant To Data(type=path "", Variant=w5457) -> (data=w5453:path)  [unwired: 1 in, 1 out]
            n2089 = call <resource>:"CommonVIs_UmlOpenVIRef.vi"("error in"=w5447) -> ("error out"=w5446:errorcluster, "AppRefOut"=w5445:refnum<vi>)  [unwired: 3 in, 6 out]
            n2090 = Open VI Reference(application reference (local)=w5445, vi path=w5453, error in (no error)=w5446) -> (vi reference=w5452:refnum<vi>, error out=w5448:errorcluster)  [unwired: 3 out]
            n2091 = property class="VI"(reference=w5452, error in=w5448, "Front Panel Window:Open"=TRUE) -> (reference out=w5450:refnum<vi>, error out=w5449:errorcluster)
            n2092 = Close Reference(reference=w5450, error in (no error)=w5449) -> (error out=w5444:errorcluster)
            n2093 = case shown="Error" w5444 {
              frame No Error {
              }
              frame Error {
                n2094 = One Button Dialog(message="The file was not possible to open with this version of LabVIEW") -> ()  [unwired: 1 in, 1 out]
              }
            }
          }
          frame "LocateInProject" {
            n2095 = call <resource>:"CommonVIs_UmlOpenVIRef.vi"("error in"=w5464) -> ("error out"=w5466:errorcluster, "ProjectNameOut"=w5465:string, "AppRefOut"=w5459:refnum<vi>)  [unwired: 3 in, 5 out]
            n2096 = Variant To Data(type=path "", Variant=w5470) -> (data=w5460:path)  [unwired: 1 in, 1 out]
            n2097 = call <resource>:"GDSProject_GetProjects.vi"("GetProjectRefByName"=w5465, "error in (no error)"=w5466) -> ("Project Refnum"=w5463:refnum<vi>, "error out"=w5462:errorcluster)  [unwired: 1 in, 15 out]
            n2098 = call <vilib>:"Get File Extension.vi"("file"=w5460) -> ("lowercase file extension"=w5461:string)  [unwired: 7 in, 3 out]
            n2099 = case shown="\"lvclass\"" w5461 {
              tunnel: w5463 -> [_ w5477 w5511 _]
              tunnel: w5462 -> [_ w5476 w5507 _]
              tunnel: w5460 -> [_ w5472 w5508 _]
              tunnel: w5459 -> [_ w5471 w5509 _]
              frame "False", Default {
              }
              frame "ctl", "vi" {
                n2100 = Open VI Reference(application reference (local)=w5471, vi path=w5472, error in (no error)=w5476) -> (vi reference=w5473:refnum<vi>, error out=w5482:errorcluster)  [unwired: 3 in]
                n2101 = invoke class="Project" method="Proj Item From Ref"(reference=w5477, error in=w5482, "VI"=w5473) -> (reference out=w5474:refnum<vi>, error out=w5481:errorcluster, "ProjItemFromRef"=w5478:refnum<vi>)  [unwired: 1 in, 1 out]
                n2102 = Not A Number/Path/Refnum?(number/path/refnum=w5478) -> (NaN/Path/Refnum?=w5479:bool)
                n2103 = Close Reference(reference=w5473, error in (no error)=w5481) -> (error out=w5480:errorcluster)
                n2104 = case shown="True" w5479 {
                  tunnel: [w5483 w5496] -> w5475
                  tunnel: w5478 -> [w5488 _]
                  tunnel: w5474 -> [w5487 w5498]
                  tunnel: w5480 -> [w5486 w5497]
                  frame False {
                    w5491 = TRUE ("Select")
                    n2105 = invoke class="Project" method="Open Window"(reference=w5487, error in=w5486) -> (error out=w5489:errorcluster)  [unwired: 1 in, 2 out]
                    n2106 = invoke class="ProjectItem" method="Make Item Visible in Tree"(reference=w5488, error in=w5489) -> (reference out=w5492:refnum<vi>, error out=w5490:errorcluster)  [unwired: 1 in, 1 out]
                    n2107 = invoke class="ProjectItem" method="SelectItem"(reference=w5492, error in=w5490, "Select"=w5491, "ClearPreviousSelection"=w5491) -> (reference out=w5485:refnum<vi>, error out=w5484:errorcluster)  [unwired: 1 in, 3 out]
                    n2108 = Close Reference(reference=w5485, error in (no error)=w5484) -> (error out=w5483:errorcluster)
                  }
                  frame True {
                    n2109 = property class="Project"(reference=w5498, error in=w5497) -> (error out=w5496:errorcluster, "Name"=w5494:string)  [unwired: 1 out]
                    n2110 = Format Into String(format string="This item: %s couldn't be found in the project" ("message"), w5494) -> (resulting string=w5493:string)  [unwired: 2 in, 1 out]
                    n2111 = One Button Dialog(message=w5493) -> ()  [unwired: 1 in, 1 out]
                  }
                }
                n2112 = Close Reference(reference=w5474, error in (no error)=w5475) -> ()  [unwired: 1 out]
              }
              frame "lvclass" {
                n2113 = invoke class="App" method="LVClass.Open"(reference=w5509, error in=w5507, "Path"=w5508) -> (error out=w5506:errorcluster, "LVClass.Open"=w5500:refnum<vi>)  [unwired: 1 in, 2 out]
                n2114 = property class="LVClassLibrary"(reference=w5500, error in=w5506) -> (error out=w5505:errorcluster, "Member Data"=w5504:refnum<vi>)  [unwired: 1 out]
                n2115 = invoke class="Project" method="Proj Item From Ref"(reference=w5511, error in=w5505, "VI"=w5504) -> (reference out=w5503:refnum<vi>, error out=w5502:errorcluster, "ProjItemFromRef"=w5512:refnum<vi>)  [unwired: 1 in, 1 out]
                n2116 = Not A Number/Path/Refnum?(number/path/refnum=w5512) -> (NaN/Path/Refnum?=w5513:bool)
                n2117 = Close Reference(reference=w5504, error in (no error)=w5502) -> (error out=w5501:errorcluster)
                n2118 = Close Reference(reference=w5500, error in (no error)=w5501) -> (error out=w5499:errorcluster)
                n2119 = case shown="False" w5513 {
                  tunnel: [w5514 w5527] -> w5510
                  tunnel: w5512 -> [w5519 _]
                  tunnel: w5503 -> [w5518 w5529]
                  tunnel: w5499 -> [w5517 w5528]
                  frame False {
                    w5522 = TRUE ("Select")
                    n2120 = invoke class="Project" method="Open Window"(reference=w5518, error in=w5517) -> (error out=w5520:errorcluster)  [unwired: 1 in, 2 out]
                    n2121 = invoke class="ProjectItem" method="Make Item Visible in Tree"(reference=w5519, error in=w5520) -> (reference out=w5523:refnum<vi>, error out=w5521:errorcluster)  [unwired: 1 in, 1 out]
                    n2122 = invoke class="ProjectItem" method="SelectItem"(reference=w5523, error in=w5521, "Select"=w5522, "ClearPreviousSelection"=w5522) -> (reference out=w5516:refnum<vi>, error out=w5515:errorcluster)  [unwired: 1 in, 3 out]
                    n2123 = Close Reference(reference=w5516, error in (no error)=w5515) -> (error out=w5514:errorcluster)
                  }
                  frame True {
                    n2124 = property class="Project"(reference=w5529, error in=w5528) -> (error out=w5527:errorcluster, "Name"=w5525:string)  [unwired: 1 out]
                    n2125 = Format Into String(format string="This item: %s couldn't be found in the project" ("message"), w5525) -> (resulting string=w5524:string)  [unwired: 2 in, 1 out]
                    n2126 = One Button Dialog(message=w5524) -> ()  [unwired: 1 in, 1 out]
                  }
                }
                n2127 = Close Reference(reference=w5503, error in (no error)=w5510) -> ()  [unwired: 1 out]
              }
              frame "lvlib" {
                n2128 = One Button Dialog(message="Function not supported yet.") -> ()  [unwired: 1 in, 1 out]
              }
            }
          }
          frame "CreateVI" {
            n2129 = Index Array(array=w5557) -> (element=w5531:refnum<class "AbstractNode.lvclass">)  [unwired: 1 in]
            n2130 = To More Specific Class(target class=refnum<class "ClassNode.lvclass"> refnum ("reference"), reference=w5531) -> (specific class reference=w5532:refnum<class "ClassNode.lvclass">)  [unwired: 1 in, 1 out]
            n2131 = call <resource>:"CommonVIs_UmlOpenVIRef.vi"() -> ("AppRefOut"=w5534:refnum<vi>)  [unwired: 4 in, 7 out]
            n2132 = call-dynamic "getClassInfo.vi"("reference"=w5532, "error in (no error)"=w5556) -> ("className"=w5554:string, "ClassPath"=w5535:path, "error out"=w5555:errorcluster)  [unwired: 8 in, 7 out]
            n2133 = call <resource>:"CommonVIs SterotypeStringParser.vi"("SterotypeStringIn"=w5554) -> ("StereoType"=w5551:T37, "Sterotype"=w5543:string)  [unwired: 17 out]
            n2134 = call <resource>:"File_ApplicationPaths.vi"("PathName"=UMLEditor_StoredPathes."ApplicationTemplatePath" ("UMLPathes")) -> ("Path Out"=w5548:path)  [unwired: 3 in, 15 out]
            n2135 = call <resource>:"File_ApplicationPaths.vi"("PathName"=UMLEditor_StoredPathes."ViTemplatePath" ("UMLPathes")) -> ("Path Out"=w5547:path)  [unwired: 3 in, 15 out]
            n2136 = Equal?(x=CommonVIs_StereoType."APPLICATION", y=w5551) -> (x = y?=w5549:bool)
            n2137 = Select(t=w5548, s=w5549, f=w5547) -> (s? t:f=w5542:path)
            n2138 = Empty String/Path?(string/path=w5542) -> (empty?=w5544:bool)
            n2139 = case shown="False" w5544 {
              tunnel: [w5566 w5571] -> w5562
              tunnel: [w5565 w5570] -> w5560
              tunnel: w5555 -> [w5564 w5569]
              tunnel: w5542 -> [_ w5568]
              tunnel: w5534 -> [w5563 w5567]
              frame True {
                n2140 = New VI(8:w5564, 11:w5563) -> (0:w5565:errorcluster, 3:w5566:refnum<vi>)  [unwired: 5 out]
              }
              frame False {
                n2141 = New VI(8:w5569, 10:w5568, 11:w5567) -> (0:w5570:errorcluster, 3:w5571:refnum<vi>)  [unwired: 4 out]
              }
            }
            n2142 = property class="VI"(reference=w5562, error in=w5560, "Front Panel Window:Open"=TRUE) -> (reference out=w5552:refnum<vi>, error out=w5553:errorcluster)
            n2143 = invoke class="VI" method="Save.Instrument"(reference=w5552, error in=w5553, "Path to saved file"=w5535) -> (reference out=w5541:refnum<vi>, error out=w5540:errorcluster)  [unwired: 3 in, 4 out]
            n2144 = Format Into String(format string="Error occurred when trying to create %s\nPath:%s\nTemplateFilePath:%s", w5543, w5535, w5542) -> (resulting string=w5545:string)  [unwired: 2 in, 1 out]
            n2145 = Close Reference(reference=w5541, error in (no error)=w5540) -> (error out=w5539:errorcluster)
            n2146 = case shown="No Error" w5539 {
              tunnel: w5545 -> [_ w5578]
              tunnel: [UMLEditor_statesType."ExecuteCommand" ("state") UMLEditor_statesType."Idle" ("state")] -> w5538
              tunnel: w5537 -> [w5573 w5576]
              tunnel: [w5574 w5576] -> w5536
              frame No Error {
                n2147 = Bundle By Name(cluster=w5573, "FlattenCommandSettings.Command"=UMLEditor_ExecuteCommandType."SyncCodeFromUML") -> (w5574:T7)
              }
              frame Error {
                n2148 = One Button Dialog(message=w5578) -> ()  [unwired: 2 out]
              }
            }
          }
          frame "SyncCodeFromUML" {
            n2149 = Index Array(array=w5581) -> (element=w5579:refnum<class "AbstractNode.lvclass">)  [unwired: 1 in]
            n2150 = call <resource>:"UMLEditor SyncCodeFromUml.vi"("error in"=w5582, "graph"=w5583, "selectedNode"=w5579) -> ("error out"=w5580:errorcluster)  [unwired: 1 in, 7 out]
          }
        }
      }
      frame "ApplyDesignPattern" {
        n2151 = Unbundle By Name(w5598) -> ("lastMousePoint"=w5587:T12, "SelectedNodes"=w5594:refnum<class "AbstractNode.lvclass">[])
        n2152 = Unbundle By Name(w5598) -> ("graphics"=w5597:refnum<class "Graphics.lvclass">, "grid"=w5596:refnum<class "Grid.lvclass">)
        n2153 = call <resource>:"UMLEditor getDiagramInfo.vi"("localVariables"=w5598, "error in (no error)"=w5600) -> ("graph"=w5595:refnum<class "Graph.lvclass">, "error out"=w5593:errorcluster)  [unwired: 16 out]
        n2154 = call <resource>:"SelectPatternDialog.vi"("GraphIn"=w5595, "SelectedNodes"=w5594, "error in"=w5593) -> ("GraphOut"=w5588:refnum<class "Graph.lvclass">, "Cancelled"=w5591:bool, "NodesOut"=w5590:T63[], "LinksOut"=w5589:T65[], "NodeIndexies"=w5586:i32[], "error out"=w5592:errorcluster)  [unwired: 11 in]
        n2155 = case shown="False" w5591 {
          tunnel: w5592 -> [w5621 w5630]
          tunnel: [w5625 w5630] -> w5601
          tunnel: w5598 -> [w5606 w5629]
          tunnel: [w5627 w5629] -> w5599
          tunnel: w5597 -> [w5622 _]
          tunnel: w5596 -> [w5623 _]
          tunnel: w5590 -> [w5618 _]
          tunnel: w5589 -> [w5617 _]
          tunnel: w5588 -> [w5624 _]
          tunnel: w5587 -> [w5616 _]
          tunnel: w5586 -> [w5607 _]
          frame False {
            n2156 = Unbundle(w5616) -> ("x"=w5614:dbl, "y"=w5609:dbl)
            n2157 = Not A Number/Path/Refnum?(number/path/refnum=w5609) -> (NaN/Path/Refnum?=w5610:bool)
            n2158 = Not A Number/Path/Refnum?(number/path/refnum=w5614) -> (NaN/Path/Refnum?=w5615:bool)
            n2159 = Select(t=0.0, s=w5610, f=w5609) -> (s? t:f=w5608:dbl)
            n2160 = Select(t=0.0, s=w5615, f=w5614) -> (s? t:f=w5612:dbl)
            n2161 = call <resource>:"DesignPatterns_DrawNodesAndLinks.vi"("GraphIn"=w5624, "Graphics"=w5622, "Grid"=w5623, "Nodes"=w5618, "Links"=w5617, "error in (no error)"=w5621, "Y-Offset"=w5608, "NodeIndexies"=w5607, "X-Offset"=w5612) -> ("GraphOut"=w5619:refnum<class "Graph.lvclass">, "NodesCreated/Modified"=w5604:refnum<class "AbstractNode.lvclass">[], "error out"=w5620:errorcluster)  [unwired: 8 in]
            n2162 = Bundle By Name(cluster=w5606, "selcted"=UMLEditor_tooltype."Node", "SelectedNodes"=w5604) -> (w5605:T7)
            n2163 = call <resource>:"UMLEditor setDiagramInfo.vi"("error in (no error)"=w5620, "localVariablesIn"=w5605, "action"=enum16{"Name/Dir", "Unsaved", "Saved"}."Unsaved") -> ("localVariablesOut"=w5627:T7, "error out"=w5626:errorcluster)  [unwired: 2 in, 13 out]
            n2164 = call-dynamic "layout.vi"("reference"=w5619, "error in (no error)"=w5626) -> ("error out"=w5625:errorcluster)  [unwired: 16 in, 1 out]
          }
          frame True {
          }
        }
      }
      frame "SyncAll" {
        n2165 = Unbundle By Name(w5632) -> ("graphics"=w5641:refnum<class "Graphics.lvclass">, "grid"=w5640:refnum<class "Grid.lvclass">)
        n2166 = call <resource>:"UMLEditor getDiagramInfo.vi"("localVariables"=w5632, "error in (no error)"=w5655) -> ("graph"=w5654:refnum<class "Graph.lvclass">, "error out"=w5644:errorcluster)  [unwired: 16 out]
        n2167 = call-dynamic "getNodes.vi"("reference"=w5654, "error in (no error)"=w5644) -> ("reference out"=w5642:refnum<class "Graph.lvclass">, "nodes"=w5649:refnum<class "AbstractNode.lvclass">[], "error out"=w5650:errorcluster)  [unwired: 15 in]
        n2168 = Index Array(array=w5649) -> (element=w5653:refnum<class "AbstractNode.lvclass">)  [unwired: 1 in]
        n2169 = Initialize Array(w5653, 0 ("dimension size")) -> (w5651:refnum<class "AbstractNode.lvclass">[])
        n2170 = local read "StatusBar"() -> (w5633:string)
        n2171 = for {
          shift-right: [w5716] -> w5639
          shift-left: w5650 -> [w5718]
          tunnel: w5649 -> [w5717] mode=indexing
          shift-right: [w5713] -> w5645
          shift-left: w5651 -> [w5715]
          n2172 = call <resource>:"AbstractNode_GetObjectStatus.vi"("reference in"=w5717, "error in (no error)"=w5718) -> ("Class name"=w5712:string, "reference out"=w5714:refnum<class "AbstractNode.lvclass">, "error out"=w5716:errorcluster)  [unwired: 15 out]
          n2173 = Match Pattern(string=w5712, regular expression="ClassNode$") -> (offset past match=w5710:i32)  [unwired: 4 out]
          n2174 = case shown="Default" w5710 {
            tunnel: w5715 -> [w5719 w5722]
            tunnel: w5714 -> [_ w5721]
            tunnel: [w5719 w5720] -> w5713
            frame -1 {
            }
            frame Default {
              n2175 = Build Array (concatenate)(w5722, w5721) -> (w5720:refnum<class "AbstractNode.lvclass">[])
            }
          }
        }
        n2176 = Equal?(x=w5637, y=UMLEditor_statesType."AutoSync") -> (x = y?=w5635:bool)
        n2177 = case shown="True" w5635 {
          frame False {
          }
          frame True {
            n2178 = property on="Picture" class="Pict"("DisabledEnum"=T38."Disabled and Grayed Out" ("Disabled")) -> (error out=w5665:errorcluster)  [unwired: 2 in, 1 out]
            n2179 = call <vilib>:"Set Busy.vi"("error in (no error)"=w5665) -> ()  [unwired: 9 in, 2 out]
          }
        }
        n2180 = for {
          N -> [w5666]
          shift-right: [w5695] -> w5634
          shift-left: w5639 -> [w5689]
          tunnel: w5645 -> [w5676] mode=indexing
          tunnel: w5642 -> [w5692]
          tunnel: w5641 -> [w5691]
          tunnel: w5640 -> [w5690]
          shift-right: [w5678] -> _
          shift-left: path[] [] -> [w5678]
          tunnel: w5635 -> [w5673]
          tunnel: w5633 -> [_]
          i -> [w5670]
          stop <- w5674 stop-if-true
          n2181 = To More Specific Class(target class=refnum<class "ClassNode.lvclass"> refnum ("reference"), reference=w5676) -> (specific class reference=w5675:refnum<class "ClassNode.lvclass">)  [unwired: 1 in, 1 out]
